vi "写入二维图片.vi"(8 "error in (no error)":errorcluster caption="错误输入（无错误）", 10 "二维图片":picture, 11 "Nagivation 2.0输入":refnum<class "Nagivation 2.0.lvclass">) -> (0 "error out":errorcluster caption="错误输出", 3 "Nagivation 2.0输出":refnum<class "Nagivation 2.0.lvclass">)   [LabVIEW 2018, in "Nagivation 2.0.lvclass"]
uses:
  Nagivation 2.0.lvclass
  Nagivation 2.0.lvclass/Nagivation 2.0.ctl
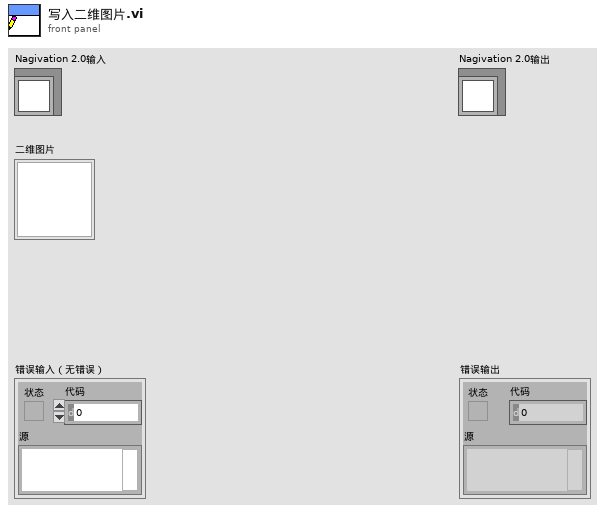
[diagram p1: front panel]
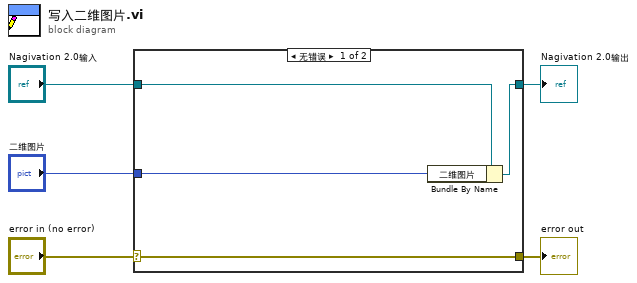
[diagram p0: block diagram]
diagram:
  n1 = case shown="无错误" "error in (no error)" {
    selector: "error in (no error)" -> [w9 w10]
    tunnel: [w9 w10] -> w4
    tunnel: [w7 w11] -> w2
    tunnel: "Nagivation 2.0输入" -> [w8 w11]
    tunnel: "二维图片" -> [w6 _]
    frame No Error {
      n2 = Bundle By Name(cluster=w8, "二维图片"=w6) -> (w7:refnum<class "Nagivation 2.0.lvclass">)
    }
    frame Error {
    }
  }
  "error out" <- w4
  "Nagivation 2.0输出" <- w2
